vi "Funcion RC.vi"() -> ()   [LabVIEW 2017]
uses:
  <vilib>/addons/System Identification/Parametric Estimation.llb/SI Estimate Continuous Transfer Function Model (SISO Array).vi
  <vilib>/addons/System Identification/NI_SysID.lvlib
panel:
  out "Waveform Chart":dbl(graph)
  in  "dt":dbl=0.01
  in  "to":dbl
  in  "tf":dbl=10.0
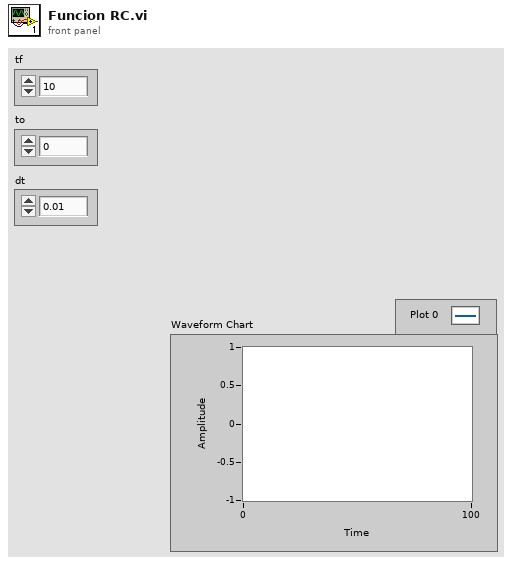
[diagram p1: front panel]
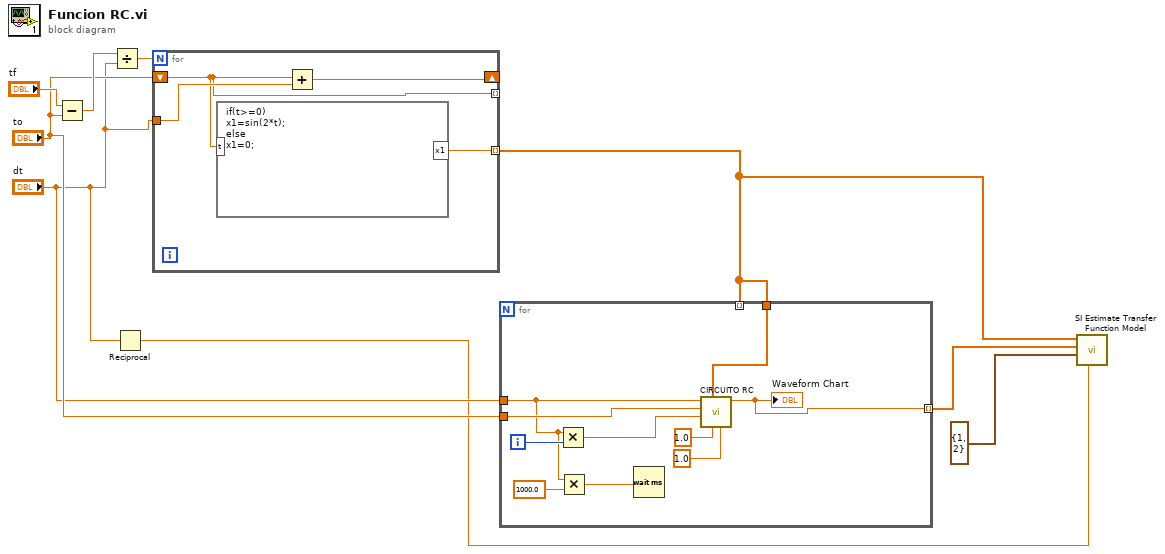
[diagram p0: block diagram]
diagram:
  n1 = Subtract(x="tf", y="to") -> (x-y=w7:dbl)
  n2 = Divide(x=w7, y="dt") -> (x/y=w8:dbl)
  n3 = Reciprocal(x="dt") -> (1/x=w1:dbl)
  n4 = for {
    N: w8 -> [_]
    tunnel: "dt" -> [w13]
    shift-right: [w12] -> _
    shift-left: "to" -> [w10]
    tunnel: [w11] -> w5 mode=indexing
    tunnel: [w10] -> _ mode=indexing
    n5 = formula code="if(t>=0)\nx1=sin(2*t);\nelse\nx1=0;"("t"=w10) -> ("x1"=w11:dbl)
    n6 = Add(x=w10, y=w13) -> (x+y=w12:dbl)
  }
  n7 = for {
    tunnel: w5 -> [_] mode=indexing
    tunnel: w5 -> [w15]
    tunnel: "to" -> [w23]
    tunnel: "dt" -> [w18]
    tunnel: [w14] -> w4 mode=indexing
    i -> [w20]
    n8 = Multiply(x=w18, y=w20) -> (x*y=w19:dbl)
    n9 = Multiply(x=w18, y=1000.0 ("x")) -> (x*y=w16:dbl)
    n10 = Wait (ms)(milliseconds to wait=w16) -> ()  [unwired: 1 out]
    n11 = call "CIRCUITO RC.vi"("C"=1.0, "R"=1.0, "Array"=w15, "t"=w19, "dt"=w23, "t0"=w18) -> ("Numeric"=w14:dbl)  [unwired: 5 in]
    "Waveform Chart" <- w14
  }
  n12 = call-poly <vilib>:"SI Estimate Transfer Function Model.vi"("sampling rate (Hz)"=w1, "orders of transfer function model"=cluster{" num order":i32, "den order":i32} {" num order"=1, "den order"=2}, "response signal"=w4, "stimulus signal"=w5) -> ()  [unwired: 4 in, 4 out]
